vi "Save Log - Single Entry.vi"(0 "reference in":refnum<class "Result Logger.lvclass">, 4 "UUT Reference":refnum<class "UUT.lvclass">, 5 "error in (no error)":errorcluster) -> (14 "reference out":refnum<class "Result Logger.lvclass">, 19 "error out":errorcluster)   [LabVIEW 2017, in "Result Logger.lvclass"]
uses:
  Result Logger.lvclass
  UUT/UUT_class/UUT.lvclass
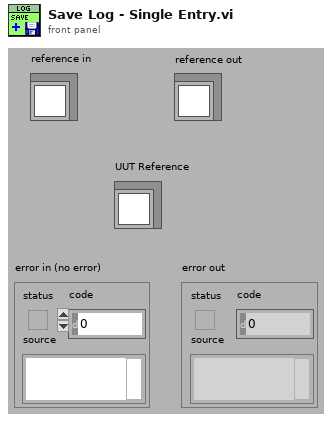
[diagram p1: front panel]
types:
  T1 = typedef "Result Logger.lvclass/ObjectAttributes.ctl" = cluster{"Logger File Path":path, "Logger File Stream":refnum<file>, "Log Messages":T2[]}
  T2 = typedef "Result Logger.lvclass/Message.ctl" = cluster{"UUT Info":cluster{"Part Number":string, "Lower Push Limit (lb)":dbl, "Upper Push Limit (lb)":dbl, "Lower Pull Limit (lb)":dbl, "Upper Pull Limit (lb)":dbl, "Push Position (mm)":dbl, "Pull Position (mm)":dbl}, "Test Results":cluster{"Test Time":timestamp, "Number of Trials":u32, "Push Values (lb)":dbl[], "Push Average (lb)":dbl, "Push Std Dev (lb)":dbl, "Push Passed":bool, "Pull Values (lb)":dbl[], "Pull Average (lb)":dbl, "Pull Std Dev (lb)":dbl, "Pull Passed":bool}}
  T3 = cluster{"Test Time":timestamp, "Number of Trials":u32, "Push Values (lb)":dbl[], "Push Average (lb)":dbl, "Push Std Dev (lb)":dbl, "Push Passed":bool, "Pull Values (lb)":dbl[], "Pull Average (lb)":dbl, "Pull Std Dev (lb)":dbl, "Pull Passed":bool}
  T4 = cluster{"Part Number":string, "Lower Push Limit (lb)":dbl, "Upper Push Limit (lb)":dbl, "Lower Pull Limit (lb)":dbl, "Upper Pull Limit (lb)":dbl, "Push Position (mm)":dbl, "Pull Position (mm)":dbl}
  T5 = cluster{"UUT Info All":cluster{"Part Number":string, "Lower Push Limit (lb)":dbl, "Upper Push Limit (lb)":dbl, "Lower Pull Limit (lb)":dbl, "Upper Pull Limit (lb)":dbl, "Push Position (mm)":dbl, "Pull Position (mm)":dbl}, "Test Results All":cluster{"Test Time":timestamp, "Number of Trials":u32, "Push Values (lb)":dbl[], "Push Average (lb)":dbl, "Push Std Dev (lb)":dbl, "Push Passed":bool, "Pull Values (lb)":dbl[], "Pull Average (lb)":dbl, "Pull Std Dev (lb)":dbl, "Pull Passed":bool}}
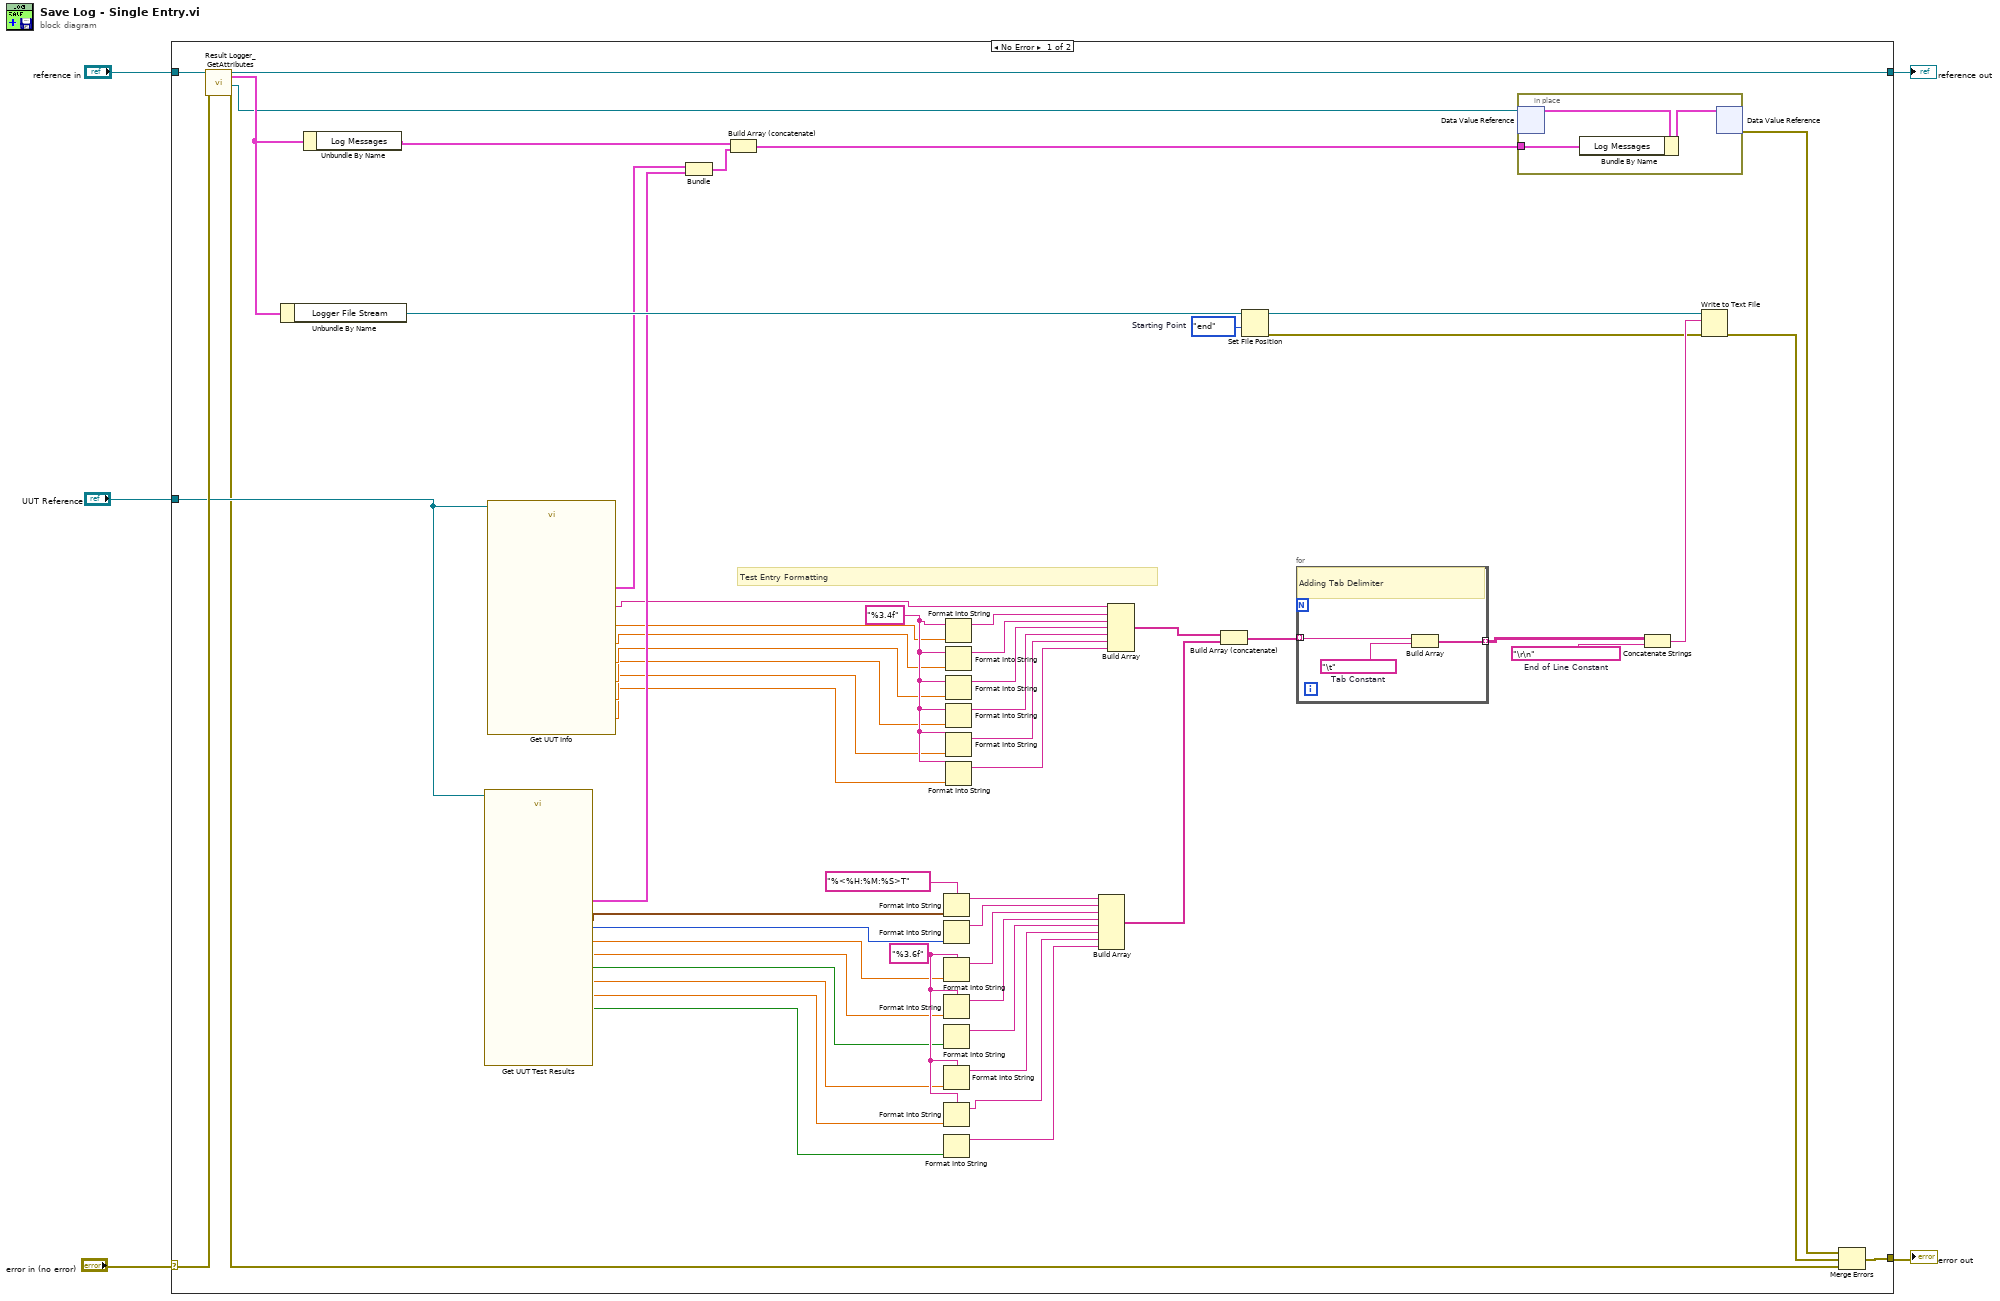
[diagram p0: block diagram]
diagram:
  n1 = case shown="No Error" "error in (no error)" {
    selector: "error in (no error)" -> [w62 w70]
    tunnel: [w8 w70] -> w4
    tunnel: [w60 w69] -> w2
    tunnel: "reference in" -> [w61 w69]
    tunnel: "UUT Reference" -> [w53 _]
    frame No Error {
      w43 = "%3.6f" ("format string")
      w45 = "%3.4f" ("format string")
      w55 = enum16{"start", "end", "current"}."end"  # Starting Point
      w54 = "\r\n"  # End of Line Constant
      # "Test Entry Formatting"
      n2 = call "Result Logger_GetAttributes.vi"("reference in"=w61, "error in (no error)"=w62) -> ("reference out"=w60:refnum<class "Result Logger.lvclass">, "Data"=w49:T1, "DataRef"=w47:refnum<data-value>, "error out"=w9:errorcluster)  [unwired: 14 in]
      n3 = Unbundle By Name(w49) -> ("Logger File Stream"=w59:refnum<file>)
      n4 = Unbundle By Name(w49) -> ("Log Messages"=w48:T2[])
      n5 = call "Get UUT Test Results.vi"("reference in"=w53) -> ("Pull Passed"=w19:bool, "Pull Std Dev (lb)"=w20:dbl, "Pull Average (lb)"=w21:dbl, "Test Results All"=w50:T3, "Test Time"=w26:timestamp, "Number of Trials"=w25:u32, "Push Average (lb)"=w24:dbl, "Push Std Dev (lb)"=w23:dbl, "Push Passed"=w22:bool)  [unwired: 14 in, 4 out]
      n6 = call "Get UUT Info.vi"("reference in"=w53) -> ("Pull Position (mm)"=w12:dbl, "UUT Info All"=w51:T4, "Push Position (mm)"=w13:dbl, "Part Number"=w18:string, "Lower Push Limit (lb)"=w17:dbl, "Upper Push Limit (lb)"=w16:dbl, "Lower Pull Limit (lb)"=w15:dbl, "Upper Pull Limit (lb)"=w14:dbl)  [unwired: 17 in, 2 out]
      n7 = Bundle("UUT Info All"=w51, "Test Results All"=w50) -> (w52:T5)  [unwired: 1 in]
      n8 = Build Array (concatenate)(w48, w52) -> (w46:T2[])
      n9 = Format Into String(format string="%<%H:%M:%S>T", w26) -> (resulting string=w36:string)  [unwired: 2 in, 1 out]
      n10 = Format Into String(w25) -> (resulting string=w35:string)  [unwired: 3 in, 1 out]
      n11 = Format Into String(format string=w43, w24) -> (resulting string=w34:string)  [unwired: 2 in, 1 out]
      n12 = Format Into String(format string=w43, w23) -> (resulting string=w33:string)  [unwired: 2 in, 1 out]
      n13 = Format Into String(w22) -> (resulting string=w32:string)  [unwired: 3 in, 1 out]
      n14 = Format Into String(format string=w43, w21) -> (resulting string=w31:string)  [unwired: 2 in, 1 out]
      n15 = Format Into String(format string=w43, w20) -> (resulting string=w30:string)  [unwired: 2 in, 1 out]
      n16 = Format Into String(w19) -> (resulting string=w29:string)  [unwired: 3 in, 1 out]
      n17 = Format Into String(format string=w45, w17) -> (resulting string=w42:string)  [unwired: 2 in, 1 out]
      n18 = Format Into String(format string=w45, w16) -> (resulting string=w41:string)  [unwired: 2 in, 1 out]
      n19 = Format Into String(format string=w45, w15) -> (resulting string=w40:string)  [unwired: 2 in, 1 out]
      n20 = Format Into String(format string=w45, w14) -> (resulting string=w39:string)  [unwired: 2 in, 1 out]
      n21 = Format Into String(format string=w45, w13) -> (resulting string=w38:string)  [unwired: 2 in, 1 out]
      n22 = Format Into String(format string=w45, w12) -> (resulting string=w37:string)  [unwired: 2 in, 1 out]
      n23 = Build Array(w36, w35, w34, w33, w32, w31, w30, w29) -> (w27:string[])
      n24 = Build Array(w18, w42, w41, w40, w39, w38, w37) -> (w28:string[])
      n25 = Build Array (concatenate)(w28, w27) -> (w7:string[])
      n26 = Set File Position(refnum=w59, from (0:start)=w55) -> (refnum out=w57:refnum<file>, error out=w56:errorcluster)  [unwired: 2 in]
      n27 = for {
        tunnel: w7 -> [w65] mode=indexing
        tunnel: [w63] -> w6 mode=indexing
        w64 = "\t"  # Tab Constant
        # "Adding Tab Delimiter"
        n28 = Build Array(w65, w64) -> (w63:string[])
      }
      n29 = in-place {
        in-place-border: w46 -> [w66]
        n30 = in-place-dvr #1(w47) -> (w67:T1)  [unwired: 1 out]
        n31 = Bundle By Name(cluster=w67, "Log Messages"=w66) -> (w68:T1)
        n32 = in-place-dvr #1(w68) -> (w11:errorcluster)  [unwired: 1 out]
      }
      n33 = Concatenate Strings(w6, w54) -> (w58:string)
      n34 = Write to Text File(file (use dialog)=w57, text=w58, error in=w56) -> (error out=w10:errorcluster)  [unwired: 1 in, 2 out]
      n35 = Merge Errors(w11, w10, w9) -> (w8:errorcluster)
    }
    frame Error {
    }
  }
  "error out" <- w4
  "reference out" <- w2
